vi "Globalclient.vi"() -> ()   [LabVIEW 2015]
panel:
  in  "通道数":enum16{"64X4", "128X4"}(ring)
  in  "connection ID 3":refnum<k5>
  out "admin?":bool
  out "Broadcast":bool
  in  "连接数":i32
  in  "未登陆":string[][](array[string])
  in  "已登陆":string[][](array[string])
  in  "CLK通道":string[][](array[string])
  out "Stop":bool
  in  "RF通道":string[][](array[string])
  in  "connection ID 2":refnum<k5>
  in  "TimeDelay":u32=100
  out "Menu":refnum<k9>
  out "PwdChecked?":bool
  out "UserName":string
  in  "connection ID":refnum<k5>
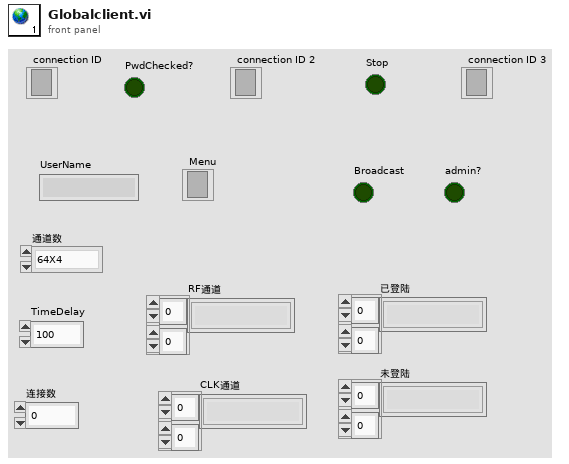
[diagram p1: front panel]
diagram:
